vi "Dock.vi"(8 "error in (no error)":errorcluster, 10 "Dock?":bool, 11 "LV MDI.lvclass":refnum<class "LV MDI.lvclass">) -> (0 "error out":errorcluster, 3 "LV MDI.lvclass":refnum<class "LV MDI.lvclass">)   [LabVIEW 2016, in "LV MDI.lvclass"]
uses:
  LV MDI.lvclass
  LV MDI.lvclass/LV MDI.ctl
  user32.dll
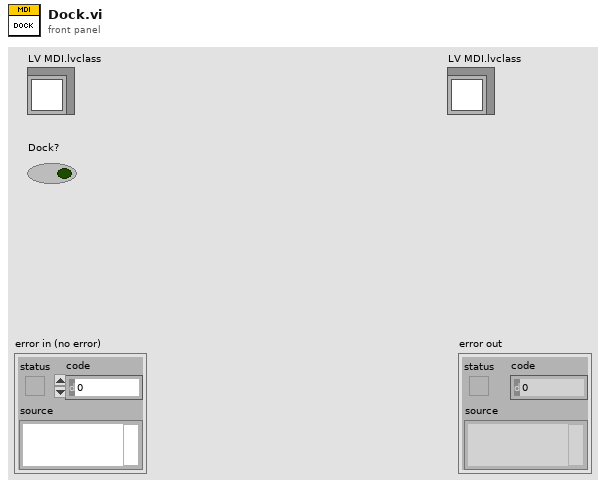
[diagram p1: front panel]
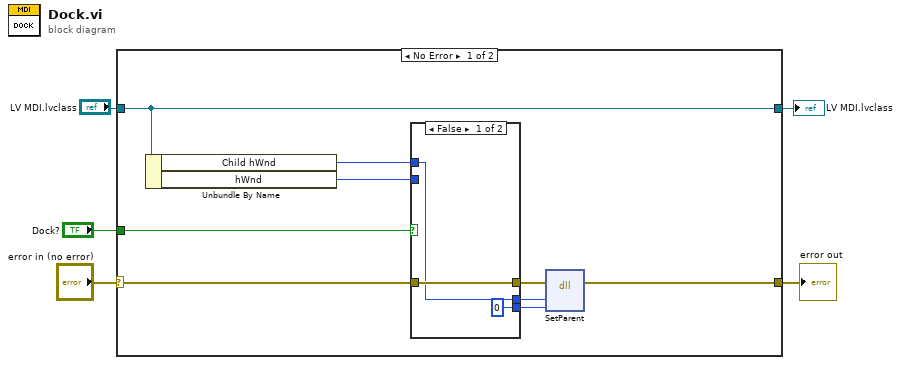
[diagram p0: block diagram]
diagram:
  n1 = case shown="No Error" "error in (no error)" {
    selector: "error in (no error)" -> [w12 w22]
    tunnel: [w13 w22] -> w4
    tunnel: [w14 w21] -> w2
    tunnel: "LV MDI.lvclass" -> [w14 w21]
    tunnel: "Dock?" -> [w10 _]
    frame No Error {
      n2 = Unbundle By Name(w14) -> ("Child hWnd"=w7:u32, "hWnd"=w6:u64)
      n3 = case shown="False" w10 {
        tunnel: w12 -> [w17 w20]
        tunnel: [w17 w20] -> w11
        tunnel: [w16 w18] -> w9
        tunnel: [u64 0 ("hWnd") w19] -> w8
        tunnel: w7 -> [w16 w18]
        tunnel: w6 -> [_ w19]
        frame False {
        }
        frame True {
        }
      }
      n4 = dll-call lib="user32.dll" fn="SetParent"(error in=w11, "Child"=w9, "NewParent"=w8) -> (error out=w13:errorcluster)  [unwired: 5 in, 1 out]
    }
    frame Error {
    }
  }
  "error out" <- w4
  "LV MDI.lvclass" <- w2
